vi "PC Take Buffer Data No Objects.vi"(7 "Photon Counter SR 400 in":T1={"Mode"=0, "Count Time"=0.0, "Trigger Frequency"=10000000.0, "Trigger External?"=FALSE, "Gate A Mode"=0, "Gate A Width"=0.0, "Gate A Delay"=0.0, "Gate B Mode"=0, "Gate B Width"=0.0, "Gate B Delay"=0.0} {"Mode" items=["A,B For T Preset", "A-B For T Preset", "A+B For T Preset", "A For B Preset"]; "Gate A Mode" items=["CW", "Fixed"]; "Gate B Mode" items=["CW", "Fixed"]}, 8 "error in (no error)":errorcluster, 11 "VISA Resource Name In":refnum<visa-resource-name>="GPIB0::23::INSTR") -> (0 "error out":errorcluster, 1 "appended array":dbl[](array[numeric]), 3 "VISA Resource Name Out":refnum<visa-resource-name>="GPIB0::23::INSTR", 5 "Photon counter SR 400 out":T1={"Mode"=0, "Count Time"=0.0, "Trigger Frequency"=10000000.0, "Trigger External?"=FALSE, "Gate A Mode"=0, "Gate A Width"=0.0, "Gate A Delay"=0.0, "Gate B Mode"=0, "Gate B Width"=0.0, "Gate B Delay"=0.0} {"Mode" items=["A,B For T Preset", "A-B For T Preset", "A+B For T Preset", "A For B Preset"]; "Gate A Mode" items=["CW", "Fixed"]; "Gate B Mode" items=["CW", "Fixed"]})   [LabVIEW 2015]
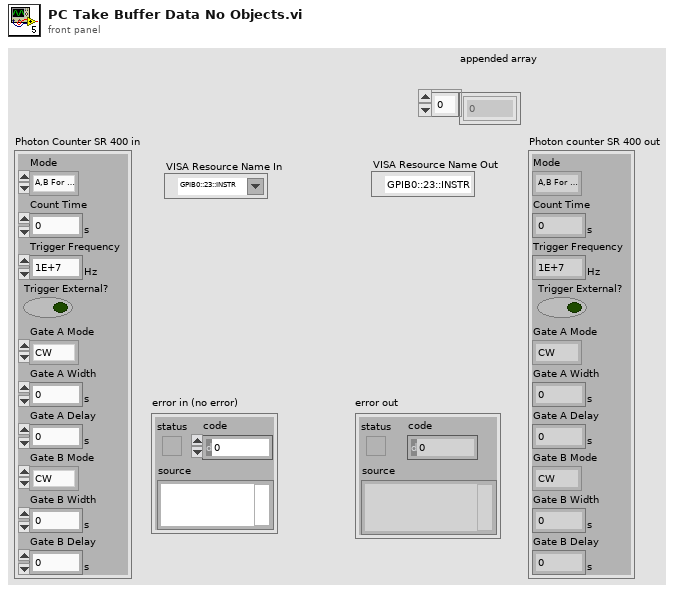
[diagram p1: front panel]
types:
  T1 = cluster{"Mode":u16, "Count Time":dbl[unit], "Trigger Frequency":dbl[unit], "Trigger External?":bool, "Gate A Mode":u16, "Gate A Width":dbl[unit], "Gate A Delay":dbl[unit], "Gate B Mode":u16, "Gate B Width":dbl[unit], "Gate B Delay":dbl[unit]}
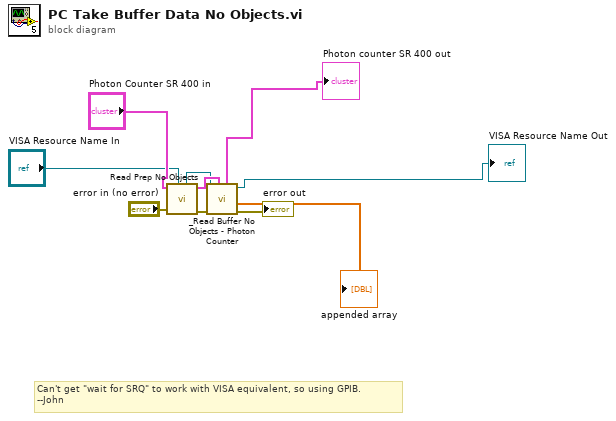
[diagram p0: block diagram]
diagram:
  # "Can't get \"wait for SRQ\" to work with VISA equivalent, so using GPIB. \n--John"
  n1 = call "Read Prep No Objects.vi"("VISA Resource Name In"="VISA Resource Name In", "error in (no error)"="error in (no error)", "Photon Counter SR 400 in"="Photon Counter SR 400 in") -> ("error out"=w5:errorcluster, "Photon Counter SR 400 out"=w7:T1, "VISA Resource Name Out"=w6:refnum<visa-resource-name>)  [unwired: 6 in]
  n2 = call "_Read Buffer No Objects - Photon Counter.vi"("Photon Counter SR 400 in"=w7, "error in (no error)"=w5, "VISA Resource Name In"=w6) -> ("error out"=→"error out":errorcluster, "appended array"=→"appended array":dbl[], "VISA Resource Name Out"=→"VISA Resource Name Out":refnum<visa-resource-name>, "Photon Counter SR 400 out"=→"Photon counter SR 400 out":T1)  [unwired: 5 in]
